vi "TTL.vi"(11 "MV":dbl(slide) scale=-100.0..100.0) -> (3 "TTL":bool[](array[boolean]))   [LabVIEW 2018]
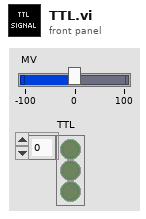
[diagram p1: front panel]
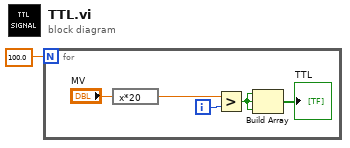
[diagram p0: block diagram]
diagram:
  n1 = for {
    N: 100.0 -> [_]
    i -> [w6]
    n2 = expression code="x*20"("MV") -> (w3:dbl)
    n3 = Greater?(x=w3, y=w6) -> (0:w5:bool)
    n4 = Build Array(w5, w5, w5) -> (→"TTL":bool[])
  }
